vi "Read E Series.vi"(8 "error in (no error)":errorcluster, 11 "file path":path) -> (0 "error out":errorcluster, 3 "E Serie Values":u16[](array[numeric]))   [LabVIEW 2018, in "E-Series Reader.lvlib"]
uses:
  E-Series Reader.lvlib
  <vilib>/Utility/file.llb/Read Delimited Spreadsheet (I64).vi
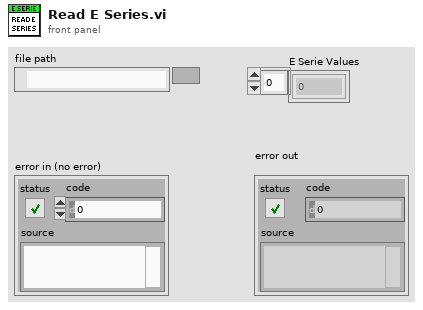
[diagram p1: front panel]
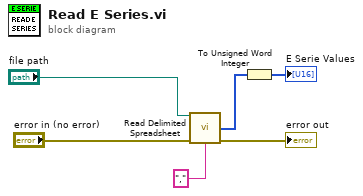
[diagram p0: block diagram]
diagram:
  n1 = call-poly <vilib>:"Read Delimited Spreadsheet.vi"("file path (dialog if empty)"="file path", "error in (no error)"="error in (no error)", "delimiter (\\t)"="," ("delimiter (\\t)")) -> ("first row"=w2:i64[], "error out"=→"error out":errorcluster)  [unwired: 7 in, 4 out]
  n2 = To Unsigned Word Integer(number=w2) -> (unsigned 16bit integer=→"E Serie Values":u16[])
